vi "Drive Direction.vi"(6 "Drive Dev Ref":T1={"DeviceStatus"={"status"=FALSE, "code"=0, "source"=""}, "Type"=enum."PWM", "PWM"={"PWM Channel"=enum."Invalid", "DeadBand"={"Name"="", "maxPositivePwm"=0, "minPositivePwm"=0, "centerPwm"=0, "maxNegativePwm"=0, "minNegativePwm"=0, "angularRange"=0}}, "CAN"={"Device Number"=0, "SetOutput VI Ref"=variant(refnum<vi> refnum), "GetOutput VI Ref"=variant(refnum<vi> refnum), "Enable VI Ref"=variant(refnum<vi> refnum), "Disable VI Ref"=variant(refnum<vi> refnum), "Data"=variant}, "Invert"=FALSE}, 7 "Swerve Dev Ref":T1={"DeviceStatus"={"status"=FALSE, "code"=0, "source"=""}, "Type"=enum."PWM", "PWM"={"PWM Channel"=enum."Invalid", "DeadBand"={"Name"="", "maxPositivePwm"=0, "minPositivePwm"=0, "centerPwm"=0, "maxNegativePwm"=0, "minNegativePwm"=0, "angularRange"=0}}, "CAN"={"Device Number"=0, "SetOutput VI Ref"=variant(refnum<vi> refnum), "GetOutput VI Ref"=variant(refnum<vi> refnum), "Enable VI Ref"=variant(refnum<vi> refnum), "Disable VI Ref"=variant(refnum<vi> refnum), "Data"=variant}, "Invert"=FALSE}, 9 "Module Number":enum16{"1", "2", "3", "4"}(ring), 10 "Wheel Power":dbl format="%#_13g", 11 "Desired direction (radians)":dbl=6.283185307179586 format="%#_13g") -> ()   [LabVIEW 2016, in "Huskie Swerve.lvlib"]
uses:
  Huskie Swerve.lvlib
  <vilib>/Rock Robotics/WPI/MotorControl/WPI_MotorControlDeviceRef.ctl
  <vilib>/Rock Robotics/WPI/MotorControl/WPI_MotorControlType.ctl
  <vilib>/Rock Robotics/SystemInterfaces/DIO/FPGA_DIOPWMChannel.ctl
  <vilib>/Rock Robotics/WPI/PWM/WPI_PWMDeadband.ctl
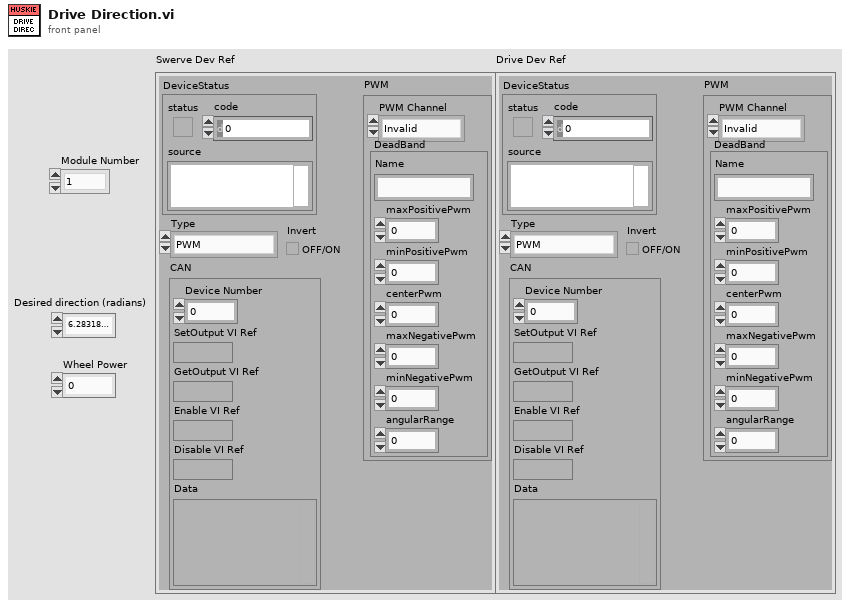
[diagram p1: front panel]
types:
  T1 = typedef "WPI_MotorControlDeviceRef.ctl" = cluster{"DeviceStatus":errorcluster, "Type":T2, "PWM":cluster{"PWM Channel":T3, "DeadBand":T4}, "CAN":cluster{"Device Number":u8, "SetOutput VI Ref":variant, "GetOutput VI Ref":variant, "Enable VI Ref":variant, "Disable VI Ref":variant, "Data":variant}, "Invert":bool}
  T2 = typedef "WPI_MotorControlType.ctl" = enum16{"PWM", "CAN"}
  T3 = typedef "FPGA_DIOPWMChannel.ctl" = enum8{"PWM 0", "PWM 1", "PWM 2", "PWM 3", "PWM 4", "PWM 5", "PWM 6", "PWM 7", "PWM 8", "PWM 9", "PWM MXP 0", "PWM MXP 1", "PWM MXP 2", "PWM MXP 3", "PWM MXP 4", "PWM MXP 5", "PWM MXP 6", "PWM MXP 7", "PWM MXP 8", "PWM MXP 9", "Invalid"}
  T4 = typedef "WPI_PWMDeadband.ctl" = cluster{"Name":string, "maxPositivePwm":i32, "minPositivePwm":i32, "centerPwm":i32, "maxNegativePwm":i32, "minNegativePwm":i32, "angularRange":u16}
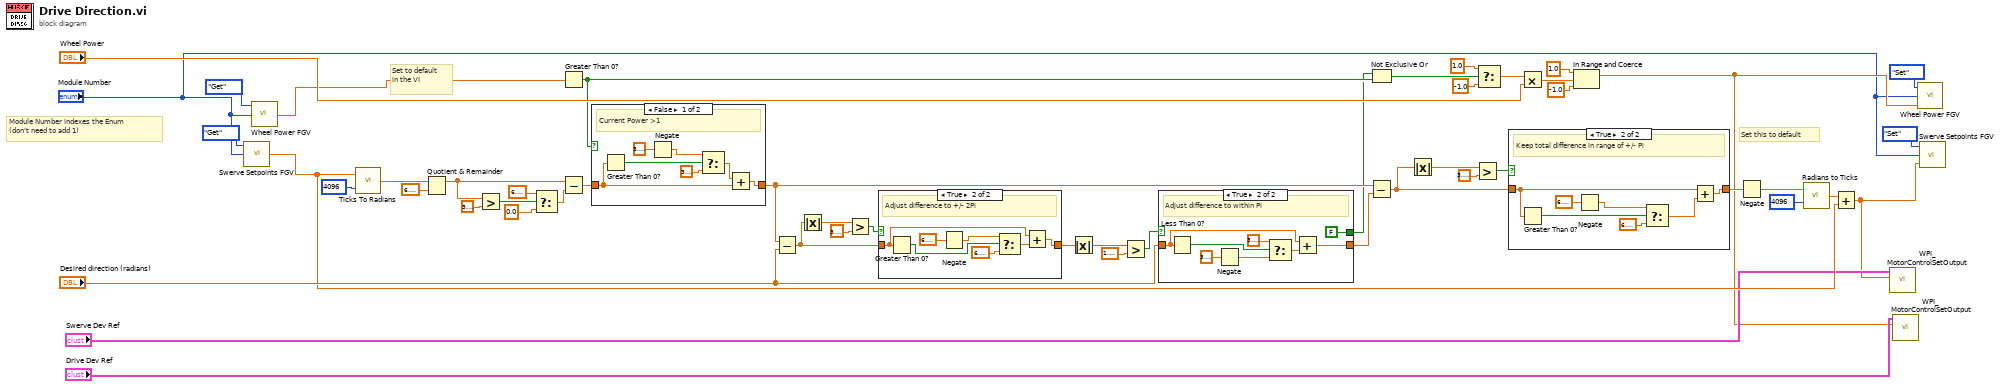
[diagram p0: block diagram]
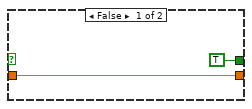
[diagram p3: hidden frame]
diagram:
  # "Module Number indexes the Enum\n(don't need to add 1)"
  # "Set this to default"
  # "Set to default\nin the VI"
  n1 = call "Swerve Setpoints FGV.vi"("Swerve Number"="Module Number", "Action"=enum16{"Set", "Get"}."Get") -> ("Setpoint"=w10:dbl)  [unwired: 1 in]
  n2 = call "Wheel Power FGV.vi"("Swerve Number"="Module Number", "Action"=enum16{"Set", "Get"}."Get") -> ("Power"=w11:dbl)  [unwired: 1 in]
  n3 = call "Ticks To Radians.vi"("Ticks/Rev"=4096, "Ticks"=w10) -> ("Radians"=w43:dbl)
  n4 = Quotient & Remainder(x=w43, y=6.283185307179586) -> (x-y*floor(x/y)=w41:dbl)  [unwired: 1 out]
  n5 = Greater?(x=w41, y=3.141592653589793) -> (0:w47:bool)
  n6 = Select(t=6.283185307179586, s=w47, f=0.0) -> (s? t:f=w44:dbl)
  n7 = Greater Than 0?(x=w11) -> (x > 0?=w13:bool)
  n8 = Subtract(x=w41, y=w44) -> (x-y=w42:dbl)
  n9 = case shown="False" w13 {
    tunnel: w42 -> [w52 w58]
    tunnel: [w51 w58] -> w25
    frame False {
      # "Current Power >1"
      n10 = Greater Than 0?(x=w52) -> (x > 0?=w57:bool)
      n11 = Negate(x=3.141592653589793) -> (-x=w56:dbl)
      n12 = Select(t=w56, s=w57, f=3.141592653589793) -> (s? t:f=w53:dbl)
      n13 = Add(x=w53, y=w52) -> (x+y=w51:dbl)
    }
    frame True {
      # "Current Power >1"
    }
  }
  n14 = Subtract(x=w25, y="Desired direction (radians)") -> (x-y=w37:dbl)
  n15 = Absolute Value(x=w37) -> (abs(x)=w38:dbl)
  n16 = Greater?(x=w38, y=3.141592653589793) -> (0:w40:bool)
  n17 = case shown="True" w40 {
    tunnel: w37 -> [w59 w61]
    tunnel: [w59 w60] -> w34
    frame False {
    }
    frame True {
      # "Adjust difference to +/- 2Pi"
      n18 = Greater Than 0?(x=w61) -> (x > 0?=w66:bool)
      n19 = Negate(x=6.283185307179586) -> (-x=w63:dbl)
      n20 = Select(t=w63, s=w66, f=6.283185307179586) -> (s? t:f=w62:dbl)
      n21 = Add(x=w61, y=w62) -> (x+y=w60:dbl)
    }
  }
  n22 = Absolute Value(x=w34) -> (abs(x)=w35:dbl)
  n23 = Greater?(x=w35, y=1.5707963267948966) -> (0:w33:bool)
  n24 = case shown="True" w33 {
    tunnel: "Desired direction (radians)" -> [w68 w71]
    tunnel: [w68 w70] -> w26
    tunnel: [TRUE FALSE] -> w12
    frame False {
    }
    frame True {
      # "Adjust difference to within Pi"
      n25 = Less Than 0?(x=w71) -> (x < 0?=w76:bool)
      n26 = Negate(x=3.141592653589793) -> (-x=w73:dbl)
      n27 = Select(t=3.141592653589793, s=w76, f=w73) -> (s? t:f=w72:dbl)
      n28 = Add(x=w71, y=w72) -> (x+y=w70:dbl)
    }
  }
  n29 = Subtract(x=w25, y=w26) -> (x-y=w28:dbl)
  n30 = Not Exclusive Or(1:w13, 2:w12) -> (0:w21:bool)
  n31 = Absolute Value(x=w28) -> (abs(x)=w31:dbl)
  n32 = Greater?(x=w31, y=3.141592653589793) -> (0:w30:bool)
  n33 = Select(t=1.0, s=w21, f=-1.0 ("t")) -> (s? t:f=w18:dbl)
  n34 = case shown="True" w30 {
    tunnel: w28 -> [w77 w79]
    tunnel: [w77 w78] -> w27
    frame False {
    }
    frame True {
      # "Keep total difference in range of +/- Pi"
      n35 = Greater Than 0?(x=w79) -> (x > 0?=w84:bool)
      n36 = Negate(x=6.283185307179586) -> (-x=w82:dbl)
      n37 = Select(t=w82, s=w84, f=6.283185307179586) -> (s? t:f=w81:dbl)
      n38 = Add(x=w79, y=w81) -> (x+y=w78:dbl)
    }
  }
  n39 = Multiply(x=w18, y="Wheel Power") -> (x*y=w14:dbl)
  n40 = In Range and Coerce(upper limit=1.0, x=w14, lower limit=-1.0) -> (coerced(x)=w7:dbl)  [unwired: 1 out]
  n41 = Negate(x=w27) -> (-x=w24:dbl)
  n42 = call "Radians to Ticks.vi"("Ticks/rev"=4096, "Radians"=w24) -> ("Ticks"=w22:dbl)
  n43 = Add(x=w22, y=w10) -> (x+y=w6:dbl)
  n44 = call <vilib>:"WPI_MotorControlSetOutput.vi"("Output"=w6, "MotorControlDevRef"="Swerve Dev Ref") -> ()  [unwired: 7 in, 3 out]
  n45 = call <vilib>:"WPI_MotorControlSetOutput.vi"("Output"=w7, "MotorControlDevRef"="Drive Dev Ref") -> ()  [unwired: 7 in, 3 out]
  n46 = call "Wheel Power FGV.vi"("New Power"=w7, "Swerve Number"="Module Number", "Action"=enum16{"Set", "Get"}."Set") -> ()  [unwired: 1 out]
  n47 = call "Swerve Setpoints FGV.vi"("New Setpoint"=w6, "Swerve Number"="Module Number", "Action"=enum16{"Set", "Get"}."Set") -> ()  [unwired: 1 out]
